vi "Really Simple Data Logger (FPGA).vi"() -> ()   [LabVIEW 2019]
uses:
  <vilib>/eio/EIONode/EIONode.xnode
  <vilib>/rvi/eio/common/nirviEmuTemplateMethod_errors.vi
panel:
  in  "AO3":fxp<+/-,20,5>
  in  "AO2":fxp<+/-,20,5>
  in  "AO1":fxp<+/-,20,5>
  out "Analog Inputs":fxp<+/-,24,5>[](array[numeric])
  in  "AO0":fxp<+/-,20,5>
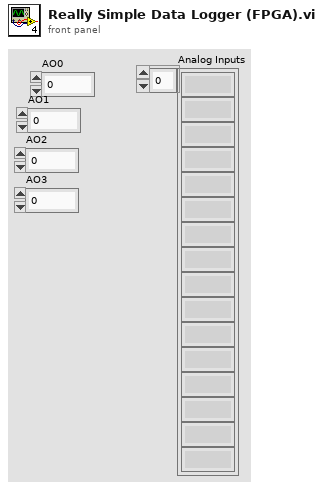
[diagram p1: front panel]
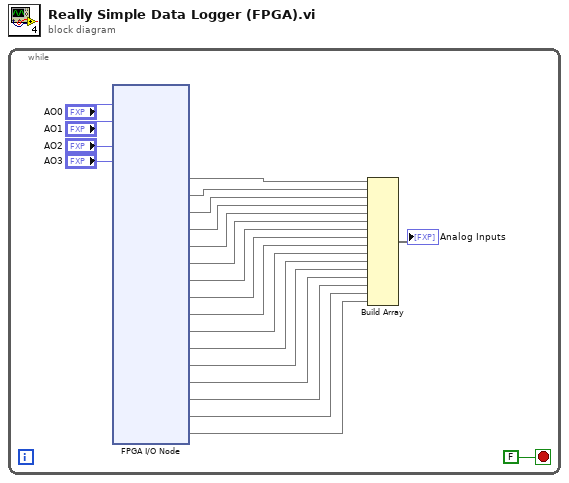
[diagram p0: block diagram]
diagram:
  n1 = while {
    stop <- FALSE stop-if-true
    n2 = xnode "FPGA I/O Node"("AO0"="AO0", "AO1"="AO1", "AO2"="AO2", "AO3"="AO3") -> ("AI0"=w21, "AI1"=w20, "AI2"=w19, "AI3"=w18, "AI4"=w17, "AI5"=w16, "AI6"=w15, "AI7"=w14, "AI8"=w13, "AI9"=w12, "AI10"=w11, "AI11"=w10, "AI12"=w9, "AI13"=w8, "AI14"=w6, "AI15"=w5)  [unwired: 20 in, 20 out]
    n3 = Build Array(w21, w20, w19, w18, w17, w16, w15, w14, w13, w12, w11, w10, w9, w8, w6, w5) -> (→"Analog Inputs":void[])
  }
